vi "Simple Channel Mapping to Channel Mapping Cluster.vi"(11 "simple channel mappings":string[](array[string])) -> (3 "channel mappings":T1[](array[typedef]))   [LabVIEW 2020, in "MeasurementServerTests.lvlib"]
uses:
  MeasurementServerTests.lvlib
  gRPC/Generated APIs/ni/measurementlink/sessionmanagement/v1/RPC Messages/ni_measurementlink_sessionmanagement_v1_ChannelMapping.ctl
  gRPC/Generated APIs/ni/measurementlink/sessionmanagement/v1/ni.measurementlink.sessionmanagement.v1.lvlib
panel:
  out "sessions":string[](array[string])
  out "instrument type ids":string[](array[string])
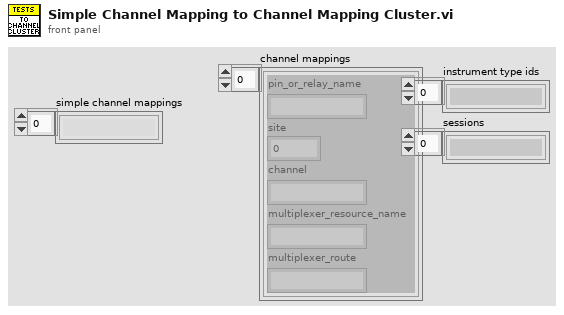
[diagram p1: front panel]
types:
  T1 = typedef "ni.measurementlink.sessionmanagement.v1.lvlib/ni_measurementlink_sessionmanagement_v1_ChannelMapping.ctl" = cluster{"pin_or_relay_name":string, "site":i32, "channel":string, "multiplexer_resource_name":string, "multiplexer_route":string}
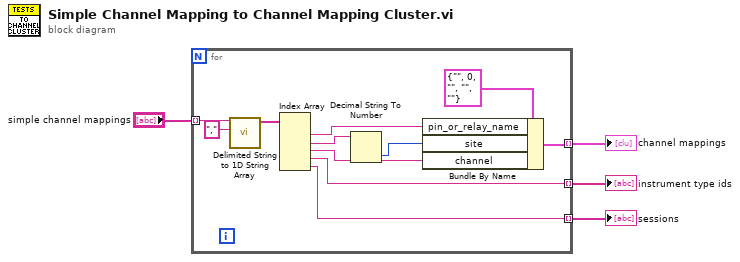
[diagram p0: block diagram]
diagram:
  n1 = for {
    tunnel: "simple channel mappings" -> [w8] mode=indexing
    tunnel: [w10] -> w4 mode=indexing
    tunnel: [w6] -> w2 mode=indexing
    tunnel: [w5] -> w1 mode=indexing
    n2 = call <vilib>:"Delimited String to 1D String Array.vi"("delimiter"=",", "delimited string"=w8) -> ("string array"=w14:string[])  [unwired: 9 in]
    n3 = Index Array(array=w14) -> (element #1=w9:string, element #2=w12:string, element #3=w13:string, element #4=w6:string, element #5=w5:string)  [unwired: 5 in]
    n4 = Decimal String To Number(string=w12) -> (number=w11:i32)  [unwired: 2 in, 1 out]
    n5 = Bundle By Name(cluster=T1 {"pin_or_relay_name"="", "site"=0, "channel"="", "multiplexer_resource_name"="", "multiplexer_route"=""} ("ni_measurementlink_sessionmanagement_v1_ChannelMapping"), "pin_or_relay_name"=w9, "site"=w11, "channel"=w13) -> (w10:T1)
  }
  "channel mappings" <- w4
  "instrument type ids" <- w2
  "sessions" <- w1
